vi "Configure Frequency.vi"(8 "error in (no error)":errorcluster, 10 "Frequency":dbl, 11 "U2000 in":refnum<class "U2000.lvclass">) -> (0 "error out":errorcluster, 3 "U2000 out":refnum<class "U2000.lvclass">)   [LabVIEW 2020, in "U2000.lvclass"]
doc: "Vi for configureting the frequency"
uses:
  U2000.lvclass
  C:/Sandbox/RF Bench/Source Code/WiSpry Test Framework/Instruments/Instrument.lvclass
  Instrument.lvclass/Instrument.ctl
  <instrlib>/Agilent U2000 Series/Agilent U2000 Series.lvlib
  Instrument.lvclass
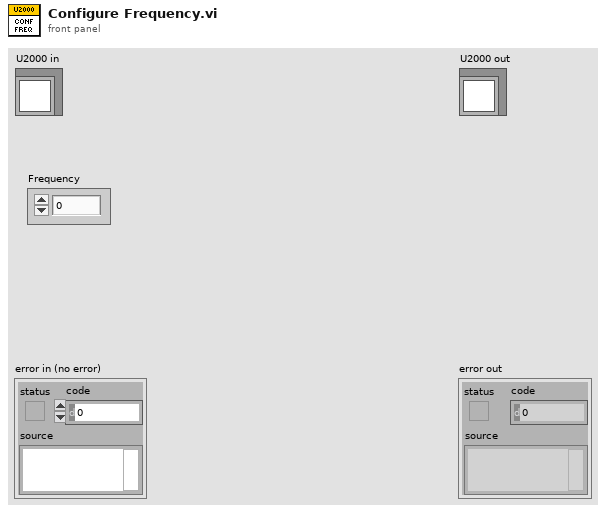
[diagram p1: front panel]
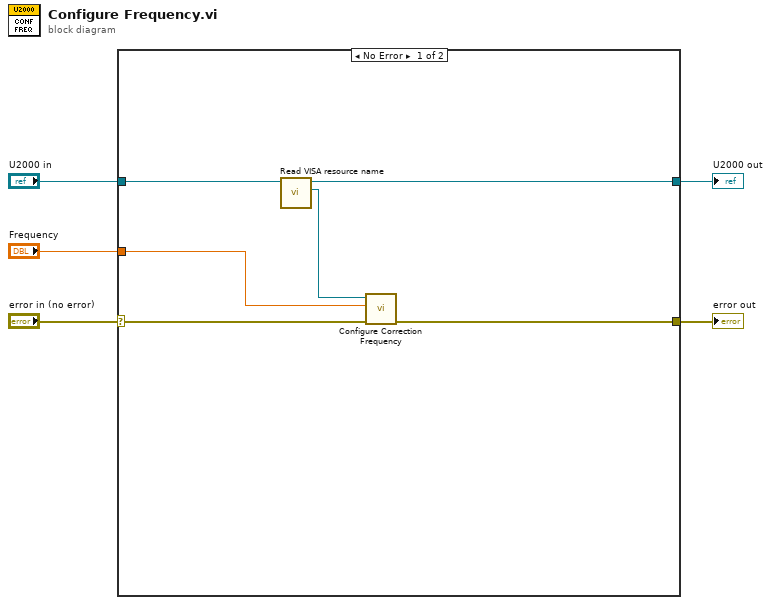
[diagram p0: block diagram]
diagram:
  n1 = case shown="No Error" "error in (no error)" {
    selector: "error in (no error)" -> [w11 w12]
    tunnel: [w10 w12] -> w5
    tunnel: [w6 w13] -> w4
    tunnel: "Frequency" -> [w9 _]
    tunnel: "U2000 in" -> [w8 w13]
    frame No Error {
      n2 = call "Read VISA resource name.vi"("Instrument in"=w8) -> ("VISA resource name"=w7:refnum<visa-resource-name>, "Instrument out"=w6:refnum<class "U2000.lvclass">)  [unwired: 9 in]
      n3 = call <instrlib>:"Configure Correction Frequency.vi"("error in (no error)"=w11, "Frequency (5E+7 Hz)"=w9, "VISA resource name"=w7) -> ("error out"=w10:errorcluster)  [unwired: 7 in, 1 out]
    }
    frame Error {
    }
  }
  "error out" <- w5
  "U2000 out" <- w4
